vi "Actor Core.vi"(8 "error in":errorcluster, 11 "Camera Settings Dialog in":refnum<class "Camera Quick Settings Panel.lvclass">) -> (0 "error out":errorcluster, 3 "Actor out":refnum<class "Actor.lvclass">)   [LabVIEW 2014, in "Camera Quick Settings Panel.lvlib" / "Camera Quick Settings Panel.lvclass"]
doc: "(<B>Filename</B>: Actor Framework.lvlib:Actor.lvclass:Actor Core.vi)\n\nReceives messages to the actor, reacts to them, and initiates any error handling that may shut the actor down.\n\nDescendant classes may override this VI to append parallel tasks for the actor to complete while it handles messages. Overrides use the Call Parent Method node."
uses:
  Camera Quick Settings Panel.lvclass
  <vilib>/ActorFramework/Actor/Actor.lvclass
  Camera Quick Settings Panel.lvclass/Camera Quick Settings Panel.ctl
  <vilib>/ActorFramework/Actor/Actor.lvclass/Actor.ctl
  <vilib>/ActorFramework/Message Enqueuer/Message Enqueuer.lvclass/Message Enqueuer.ctl
  <vilib>/ActorFramework/Message Enqueuer/Init from Existing Queue.vi
  <vilib>/ActorFramework/Message Enqueuer/Enqueue.vi
  <vilib>/ActorFramework/Message Priority Queue/Priority Enqueue.vi
  <vilib>/ActorFramework/Message Enqueuer/Message Enqueuer.lvclass
  Camera Quick Settings Panel Messages/Set Exp Time Abs Msg/Set Exp Time Abs Msg.lvclass
  Camera Quick Settings Panel Messages/Set Exposure Timebase Msg/Set Exposure Timebase Msg.lvclass
  Camera Quick Settings Panel Messages/Set Trigger Mode Msg/Set Trigger Mode Msg.lvclass
  <vilib>/ActorFramework/Stop Msg/Stop Msg.lvclass
  Shared Code/Viewable Actor/ViewableActor/ViewableActor.lvclass
panel:
  in  "Trigger":u32(ring) items=["Use hardware value", "10-bit", "12-bit", "14-bit", "16-bit"]
  in  "Timebase":dbl(slide) min=17.00000029813964 max=5000000.0 step=1.0 scale=17.00000029813964..5000000.0
  in  "Exp Time":dbl(slide) min=17.00000029813964 max=5000000.0 step=1.0 scale=17.00000029813964..5000000.0
  in  "Stop Signal":bool=TRUE
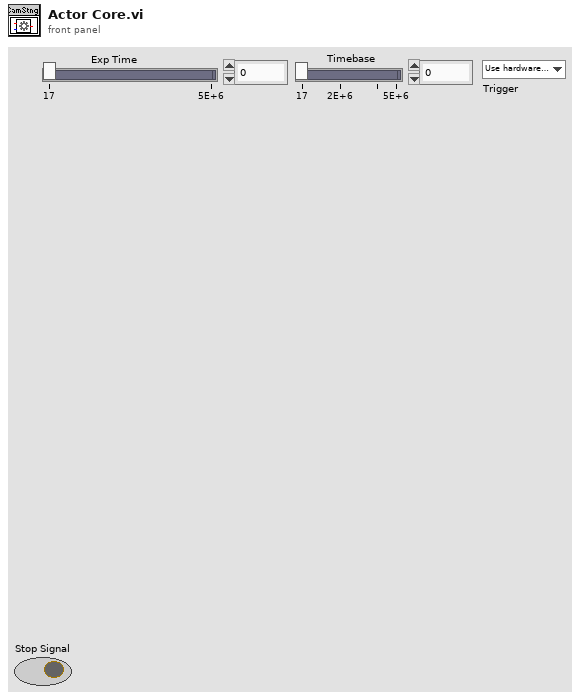
[diagram p1: front panel]
types:
  T1 = typedef "IMAQdx.ctl" = refnum<k21>
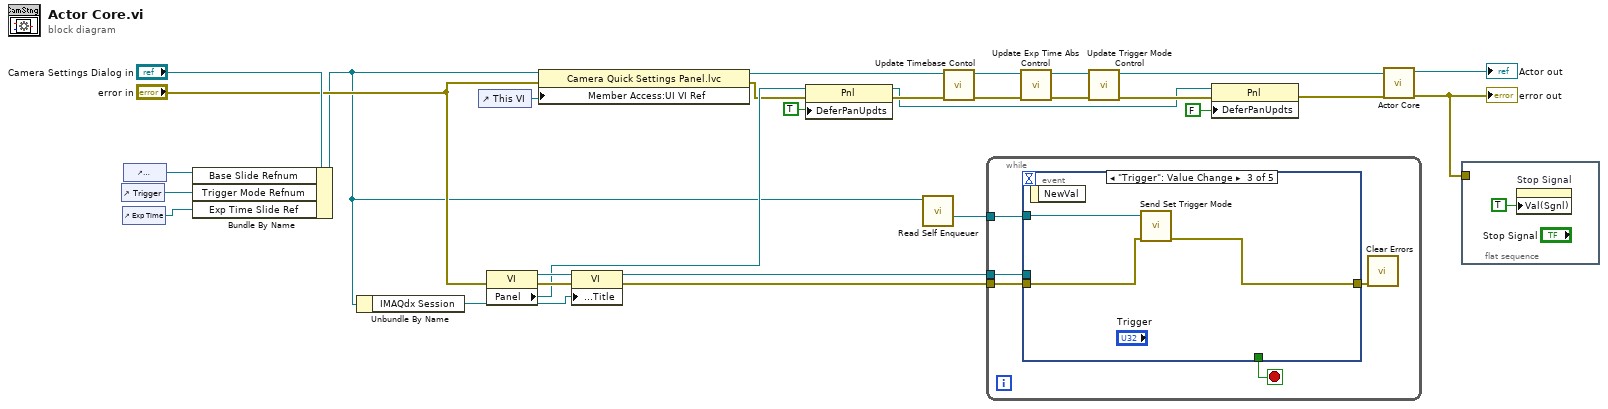
[diagram p0: block diagram]
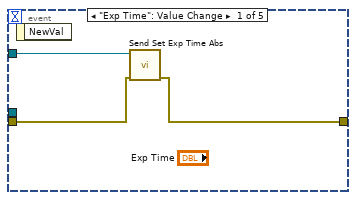
[diagram p2: hidden frame]
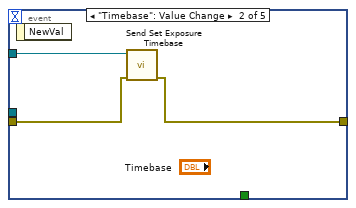
[diagram p3: hidden frame]
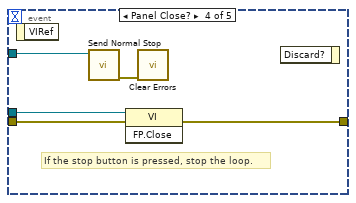
[diagram p4: hidden frame]
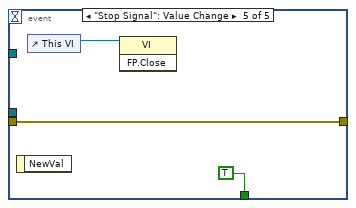
[diagram p5: hidden frame]
diagram:
  n1 = control-ref of="Trigger"() -> (w12:refnum<vi>)
  n2 = control-ref of="Exp Time"() -> (w11:refnum<vi>)
  n3 = control-ref of="Timebase"() -> (w13:refnum<vi>)
  n4 = Bundle By Name(cluster="Camera Settings Dialog in", "Base Slide Refnum"=w13, "Trigger Mode Refnum"=w12, "Exp Time Slide Ref"=w11) -> (w14:refnum<class "Camera Quick Settings Panel.lvclass">)
  n5 = Unbundle By Name(w14) -> ("IMAQdx Session"=w18:T1)
  n6 = control-ref of="This VI"() -> (w20:refnum<vi>)
  n7 = property class="VI"(error in="error in") -> (reference out=w25:refnum<vi>, error out=w27:errorcluster, "Panel"=w17:refnum<vi>)  [unwired: 1 in]
  n8 = property class="Camera Quick Settings Panel.lvc"(reference=w14, error in="error in", "Member Access:UI VI Ref"=w20) -> (reference out=w21:refnum<class "Camera Quick Settings Panel.lvclass">, error out=w10:errorcluster)
  n9 = property class="VI"(reference=w25, error in=w27, "Front Panel.Title"=w18) -> (reference out=w26:refnum<vi>, error out=w24:errorcluster)
  n10 = property class="Pnl"(reference=w17, error in=w10, "DeferPanUpdts"=TRUE ("Defer Panel Updates")) -> (reference out=w1:refnum<vi>, error out=w6:errorcluster)
  n11 = call <vilib>:"Read Self Enqueuer.vi"("Actor"=w14) -> ("Self Enqueuer"=w22:refnum<class "Message Enqueuer.lvclass">)  [unwired: 10 in]
  n12 = call-dynamic "Update Timebase Contol.vi"("error in (no error)"=w6, "Camera Quick Settings Panel in"=w21) -> ("error out"=w5:errorcluster, "Camera Quick Settings Panel out"=w9:refnum<class "Camera Quick Settings Panel.lvclass">)  [unwired: 8 in]
  n13 = while {
    tunnel: w24 -> [w34]
    tunnel: w26 -> [w32]
    tunnel: w22 -> [w30]
    stop <- w33 stop-if-true
    n14 = event shown="[2] \"Trigger\": Value Change" {
      selector: _ -> [_ _ _ _ _]
      dyn-events: _ -> [_ _ _ _ _]
      timeout: _ -> [_ _ _ _ _]
      tunnel: w34 -> [w36 w39 w42 w44 w49]
      tunnel: [w35 w38 w41 w47 w49] -> w31
      tunnel: [_ _ _ _ TRUE ("stop")] -> w33
      tunnel: w32 -> [_ _ _ w48 _]
      tunnel: w30 -> [w37 w40 w43 w46 _]
      event "Exp Time": Value Change {
        n15 = event-data() -> ()  [unwired: 2 out]
        n16 = call "Send Set Exp Time Abs.vi"("error in (no error)"=w36, "Message Enqueuer"=w37) -> ("error out"=w35:errorcluster)  [unwired: 8 in, 1 out]
      }
      event "Timebase": Value Change {
        n17 = event-data() -> ()  [unwired: 2 out]
        n18 = call "Send Set Exposure Timebase.vi"("error in (no error)"=w39, "Message Enqueuer"=w40) -> ("error out"=w38:errorcluster)  [unwired: 8 in, 1 out]
      }
      event "Trigger": Value Change {
        n19 = event-data() -> ()  [unwired: 2 out]
        n20 = call "Send Set Trigger Mode.vi"("error in (no error)"=w42, "Message Enqueuer"=w43) -> ("error out"=w41:errorcluster)  [unwired: 8 in, 1 out]
      }
      event Panel Close? {
        # "If the stop button is pressed, stop the loop."
        n21 = event-data() -> ()  [unwired: 2 out]
        n22 = call <vilib>:"Send Normal Stop.vi"("Message Enqueuer"=w46) -> ("error out"=w45:errorcluster)  [unwired: 10 in]
        n23 = invoke class="VI" method="FP.Close"(reference=w48, error in=w44) -> (error out=w47:errorcluster)  [unwired: 1 in, 2 out]
        n24 = call <vilib>:"Clear Errors.vi"("error in (no error)"=w45) -> ()  [unwired: 5 in, 2 out]
        n25 = event-data() -> ()  [unwired: 2 in, 1 out]
      }
      event "Stop Signal": Value Change {
        n26 = event-data() -> ()  [unwired: 2 out]
        n27 = control-ref of="This VI"() -> (w50:refnum<vi>)
        n28 = invoke class="VI" method="FP.Close"(reference=w50) -> ()  [unwired: 2 in, 3 out]
      }
    }
    n29 = call <vilib>:"Clear Errors.vi"("error in (no error)"=w31) -> ()  [unwired: 5 in, 2 out]
  }
  n30 = call-dynamic "Update Exp Time Abs Control.vi"("error in (no error)"=w5, "Camera Quick Settings Panel in"=w9) -> ("error out"=w4:errorcluster, "Camera Quick Settings Panel out"=w8:refnum<class "Camera Quick Settings Panel.lvclass">)  [unwired: 8 in]
  n31 = call-dynamic "Update Trigger Mode Control.vi"("error in (no error)"=w4, "Camera Quick Settings Panel in"=w8) -> ("error out"=w3:errorcluster, "Camera Quick Settings Panel out"=w7:refnum<class "Camera Quick Settings Panel.lvclass">)  [unwired: 8 in]
  n32 = property class="Pnl"(reference=w1, error in=w3, "DeferPanUpdts"=FALSE ("Defer Panel Updates")) -> (error out=w2:errorcluster)  [unwired: 1 out]
  n33 = call-parent "Actor Core.vi"("error in"=w2, "Actor in"=w7) -> ("error out"=w23:errorcluster, "Actor out"=→"Actor out":refnum<class "Actor.lvclass">)  [unwired: 8 in]
  "error out" <- w23
  n34 = flat-sequence {
    tunnel: w23 -> [_]
    frame #0 {
      n35 = property on="Stop Signal" class="Bool (strict)"("Val(Sgnl)"=TRUE) -> ()  [unwired: 2 in, 2 out]
    }
  }
